vi "divide_by_scalar.vi"(8 "error in (no error)":errorcluster, 10 "divisor":dbl=1.0, 11 "SpaceVector in":refnum<class "SpaceVector.lvclass">) -> (0 "error out":errorcluster, 3 "SpaceVector out":refnum<class "SpaceVector.lvclass">)   [LabVIEW 2010, in "SpaceVector.lvclass"]
uses:
  SpaceVector.lvclass
  SpaceVector.lvclass/SpaceVector.ctl
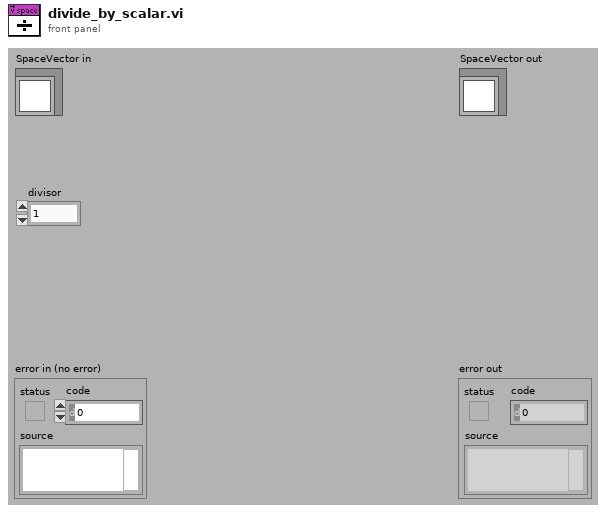
[diagram p1: front panel]
types:
  T1 = typedef "space_vector_array.ctl" = dbl[unit][]
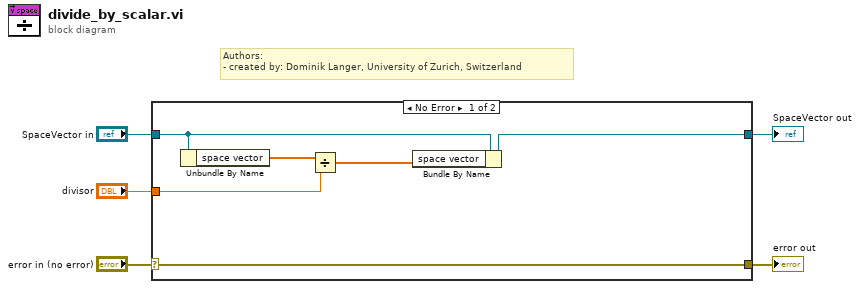
[diagram p0: block diagram]
diagram:
  # "Authors: \n- created by: Dominik Langer, University of Zurich, Switzerland"
  n1 = case shown="No Error" "error in (no error)" {
    selector: "error in (no error)" -> [w11 w13]
    tunnel: [w11 w13] -> w4
    tunnel: [w6 w12] -> w2
    tunnel: "SpaceVector in" -> [w7 w12]
    tunnel: "divisor" -> [w9 _]
    frame No Error {
      n2 = Unbundle By Name(w7) -> ("space vector"=w10:T1)
      n3 = Divide(x=w10, y=w9) -> (x/y=w8:T1)
      n4 = Bundle By Name(cluster=w7, "space vector"=w8) -> (w6:refnum<class "SpaceVector.lvclass">)
    }
    frame Error {
    }
  }
  "error out" <- w4
  "SpaceVector out" <- w2
